vi "Send Event.vi"(0 "State":T1={"Prompt"="Click to add", "Listbox"=refnum, "events"={"Items Changed"=refnum, "List Changed"=refnum}, "allow move"=FALSE}, 5 "action":T3, 7 "Name":string, 9 "Row":i32, 11 "error in (no error)":errorcluster) -> (4 "State thru":T1={"Prompt"="Click to add", "Listbox"=refnum, "events"={"Items Changed"=refnum, "List Changed"=refnum}, "allow move"=FALSE}, 15 "error out":errorcluster)   [LabVIEW 2020, in "KListbox.xctl"]
uses:
  KListbox.xctl
  Event Action.ctl
  State.ctl
  Events.ctl
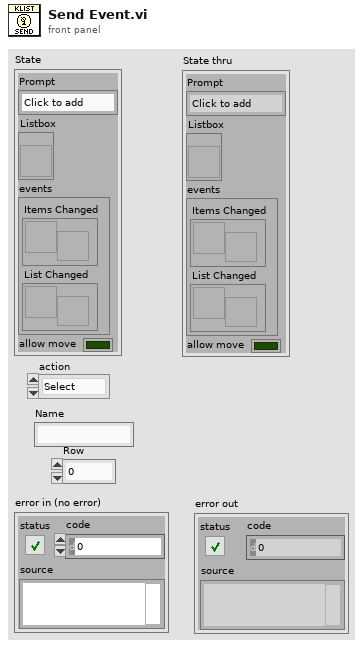
[diagram p1: front panel]
types:
  T1 = typedef "KListbox.xctl/State.ctl" = cluster{"Prompt":string, "Listbox":refnum<vi>, "events":T2, "allow move":bool}
  T2 = typedef "KListbox.xctl/Events.ctl" = cluster{"Items Changed":refnum<user-event>, "List Changed":refnum<user-event>}
  T3 = typedef "KListbox.xctl/Event Action.ctl" = enum16{"Select", "Add", "Delete", "Edit"}
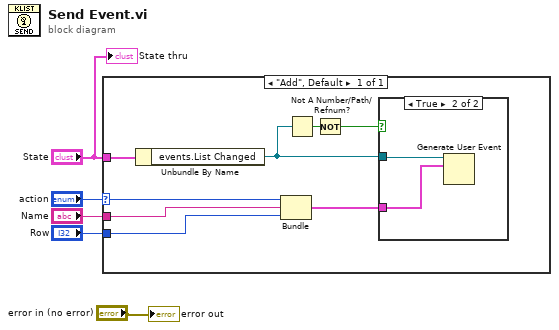
[diagram p0: block diagram]
diagram:
  n1 = case shown="\"Add\", Default" "action" {
    selector: "action" -> [w10]
    tunnel: "Name" -> [w9]
    tunnel: "Row" -> [w8]
    tunnel: "State" -> [w6]
    frame "Add", Default {
      n2 = Unbundle By Name(w6) -> ("events.List Changed"=w12:refnum<user-event>)
      n3 = Bundle("action"=w10, "Name"=w9, "Row"=w8) -> (w7:cluster{"action":T3, "Name":string, "Row":i32})  [unwired: 1 in]
      n4 = Not A Number/Path/Refnum?(number/path/refnum=w12) -> (NaN/Path/Refnum?=w13:bool)
      n5 = Not(x=w13) -> (.not. x?=w11:bool)
      n6 = case shown="True" w11 {
        tunnel: w12 -> [_ w14]
        tunnel: w7 -> [_ w15]
        frame False {
        }
        frame True {
          n7 = Generate User Event(user event=w14, event data cluster=w15) -> ()  [unwired: 2 in, 2 out]
        }
      }
    }
  }
  "error out" <- "error in (no error)"
  "State thru" <- "State"
